vi "Boolean Reset.vi"(11 "Auto Commands in":bool[](array[boolean])) -> (3 "Auto Commands out":bool[](array[boolean]))   [LabVIEW 2018]
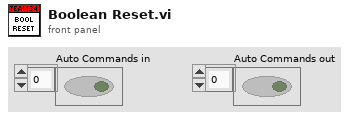
[diagram p1: front panel]
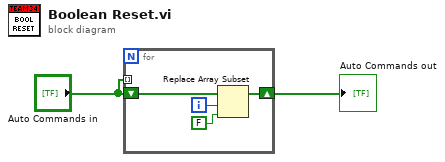
[diagram p0: block diagram]
diagram:
  n1 = for {
    tunnel: "Auto Commands in" -> [_] mode=indexing
    shift-right: [w3] -> w2
    shift-left: "Auto Commands in" -> [w6]
    i -> [w4]
    n2 = Replace Array Subset(array=w6, new element=FALSE ("new element/subarray"), index=w4) -> (w3:bool[])
  }
  "Auto Commands out" <- w2
